vi "log analysis_gps.vi"() -> ()   [LabVIEW 2019] (continued)
0.0780,0.0969,0.1020,4.9076,0f000001,0*84139aa4\n\tsystem status\tnormal 2 27.900000 0 0\trobot status\t209.409703\t112.091356\t7.992300\t-0.536108\t-0.972920\t165.803914\t0.366000\t-0.087000\n\t\n15:41:04.9\tlog_raw\tgps_raw\t#INSPVAXA,USB3,0,46.5,FINESTEERING,2107,283282.900,02000000,471d,15824;INS_ALIGNMENT_COMPLETE,INS_RTKFIXED,37.37114058950,126.72319773387,7.9934,22.3000,0.0877,-0.2549,-0.0017,-0.494597000,-1.027505059,284.193699640,0.4479,0.2971,0.5695,0.1142,0.0928,0.0780,0.0969,0.1020,4.9076,0f000001,0*ecacd8f3\n\tsystem status\tnormal 2 27.900000 0 0\trobot status\t209.277787\t112.135444\t7.993400\t-0.494597\t-1.027505\t165.806300\t0.258000\t0.054000\n\t\n15:41:05.4\tlog_raw\tgps_raw\t\tsystem status\tnormal 2 27.900000 0 0\trobot status\t209.151815\t112.177150\t7.994600\t-0.569552\t-1.072991\t165.805716\t0.270000\t0.034000\n\t\n15:41:05.9\tlog_raw\tgps_raw\t\tsystem status\tnormal 2 27.900000 0 0\trobot status\t209.015709\t112.223223\t7.996800\t-0.645711\t-1.000745\t165.770418\t0.298000\t0.003000\n\t\n15:41:06.4\tlog_raw\tgps_raw\t#INSPVAXA,USB3,0,45.5,FINESTEERING,2107,283284.400,02000000,471d,15824;INS_ALIGNMENT_COMPLETE,INS_RTKFIXED,37.37114183564,126.72319312332,7.9966,22.3000,0.0813,-0.2603,0.0021,-0.541869353,-0.903555569,284.232610240,0.4477,0.2970,0.5694,0.1142,0.0928,0.0780,0.0969,0.1020,4.9102,0f000001,0*cca71bea\n\tsystem status\tnormal 2 27.900000 0 0\trobot status\t208.869392\t112.273757\t7.996600\t-0.541869\t-0.903556\t165.767390\t0.362000\t-0.089000\n\t\n15:41:06.9\tlog_raw\tgps_raw\t\tsystem status\tnormal 2 27.900000 0 0\trobot status\t208.748375\t112.316292\t7.995100\t-0.425843\t-0.804427\t165.786468\t0.277000\t0.029000\n\t\n15:41:07.4\tlog_raw\tgps_raw\t#INSPVAXA,USB3,0,48.5,FINESTEERING,2107,283285.400,02000000,471d,15824;INS_ALIGNMENT_COMPLETE,INS_RTKFIXED,37.37114271022,126.72319003823,7.9928,22.3000,0.0833,-0.2558,0.0046,-0.428723996,-1.048111002,284.209543070,0.4481,0.2971,0.5696,0.1142,0.0929,0.0780,0.0969,0.1020,4.9114,0f000001,0*c956834d\n\tsystem status\tnormal 2 27.900000 0 0\trobot status\t208.596120\t112.370829\t7.992800\t-0.428724\t-1.048111\t165.790457\t0.290000\t0.012000\n\t\n15:41:07.9\tlog_raw\tgps_raw\t\tsystem status\tnormal 2 27.900000 0 0\trobot status\t208.491998\t112.410695\t7.991800\t-0.503839\t-1.117557\t165.853585\t0.272000\t-0.014000\n\t\n15:41:08.4\tlog_raw\tgps_raw\t\tsystem status\tnormal 2 27.900000 0 0\trobot status\t208.354984\t112.461159\t7.990800\t-0.430331\t-1.222643\t165.896888\t0.242000\t0.064000\n\t\n15:41:08.9\tlog_raw\tgps_raw\t\tsystem status\tnormal 2 27.900000 0 0\trobot status\t208.213933\t112.512805\t7.989100\t-0.303789\t-1.363039\t165.889884\t0.281000\t0.011000\n\t\n15:41:09.4\tlog_raw\tgps_raw\t\tsystem status\tnormal 2 27.900000 0 0\trobot status\t208.079726\t112.560978\t7.988900\t-0.312448\t-1.099711\t166.040201\t0.268000\t0.063000\n\t\n15:41:09.9\tlog_raw\tgps_raw\t#INSPVAXA,USB3,0,48.5,FINESTEERING,2107,283287.900,02000000,471d,15824;INS_ALIGNMENT_COMPLETE,INS_RTKFIXED,37.37114488961,126.72318257858,7.9892,22.3000,0.0816,-0.2710,-0.0129,-0.307821910,-0.791572472,283.812578734,0.4475,0.2971,0.5695,0.1142,0.0928,0.0780,0.0969,0.1020,4.9139,0f000001,0*ad245747\n\tsystem status\tnormal 2 27.900000 0 0\trobot status\t207.935356\t112.612724\t7.989200\t-0.307822\t-0.791572\t166.187421\t0.253000\t0.089000\n\t\n15:41:10.4\tlog_raw\tgps_raw\t\tsystem status\tnormal 2 27.900000 0 0\trobot status\t207.818109\t112.654789\t7.987300\t-0.128529\t-0.454330\t166.386533\t0.238000\t0.094000\n\t\n15:41:10.9\tlog_raw\tgps_raw\t\tsystem status\tnormal 2 27.900000 0 0\trobot status\t207.682381\t112.702193\t7.985100\t0.008586\t-0.367132\t166.647704\t0.354000\t-0.072000\n\t\n15:41:11.4\tlog_raw\tgps_raw\t\tsystem status\tnormal 2 27.900000 0 0\trobot status\t207.545944\t112.748506\t7.983500\t-0.104519\t-0.407601\t166.876689\t0.236000\t0.094000\n\t\n15:41:11.9\tlog_raw\tgps_raw\t\tsystem status\tnormal 2 27.900000 0 0\trobot status\t207.410608\t112.793821\t7.982300\t-0.272687\t-0.577637\t167.093526\t0.359000\t-0.081000\n\t\n15:41:12.4\tlog_raw\tgps_raw\t#INSPVAXA,USB3,0,49.0,FINESTEERING,2107,283290.400,02000000,471d,15824;INS_ALIGNMENT_COMPLETE,INS_RTKFIXED,37.37114696201,126.72317494055,7.9797,22.3000,0.0686,-0.2611,-0.0031,-0.360570478,-0.610945799,282.620180984,0.4490,0.2972,0.5701,0.1142,0.0929,0.0781,0.0969,0.1020,4.9167,0f000001,0*1d53d3bd\n\tsystem status\tnormal 2 27.800000 0 0\trobot status\t207.258792\t112.842745\t7.979700\t-0.360570\t-0.610946\t167.379819\t0.257000\t0.055000\n\t\n15:41:12.9\tlog_raw\tgps_raw\t\tsystem status\tnormal 2 27.900000 0 0\trobot status\t207.133471\t112.884794\t7.976400\t-0.101922\t-0.587644\t167.621248\t0.377000\t-0.109000\n\t\n15:41:13.4\tlog_raw\tgps_raw\t#INSPVAXA,USB3,0,45.5,FINESTEERING,2107,283291.400,02000000,471d,15824;INS_ALIGNMENT_COMPLETE,INS_RTKFIXED,37.37114777556,126.72317182162,7.9735,22.3000,0.0763,-0.2712,-0.0094,-0.152974893,-0.616653887,282.239897550,0.4489,0.2971,0.5701,0.1142,0.0928,0.0781,0.0969,0.1020,4.9171,0f000001,0*c60dfbfa\n\tsystem status\tnormal 2 27.900000 0 0\trobot status\t206.982522\t112.933044\t7.973500\t-0.152975\t-0.616654\t167.760102\t0.226000\t0.111000\n\t\n15:41:13.9\tlog_raw\tgps_raw\t\tsystem status\tnormal 2 27.900000 0 0\trobot status\t206.858547\t112.972720\t7.970000\t-0.152145\t-0.757539\t167.961795\t0.320000\t-0.033000\n\t\n15:41:14.4\tlog_raw\tgps_raw\t\tsystem status\tnormal 2 27.900000 0 0\trobot status\t206.718471\t113.014805\t7.968100\t-0.313258\t-0.816536\t168.090661\t0.278000\t0.044000\n\t\n15:41:14.9\tlog_raw\tgps_raw\t#INSPVAXA,USB3,0,45.0,FINESTEERING,2107,283292.900,02008000,471d,15824;INS_ALIGNMENT_COMPLETE,INS_RTKFIXED,37.37114893041,126.72316711689,7.9673,22.3000,0.0793,-0.2669,-0.0229,-0.307538430,-0.866474135,281.723711903,0.4489,0.2972,0.5701,0.1141,0.0929,0.0781,0.0969,0.1020,4.9176,0f000001,0*1a68f6c8\n\tsystem status\tnormal 2 27.900000 0 0\trobot status\t206.565785\t113.061225\t7.967300\t-0.307538\t-0.866474\t168.276288\t0.236000\t0.105000\n\t\n15:41:15.4\tlog_raw\tgps_raw\t#INSPVAXA,USB3,0,46.5,FINESTEERING,2107,283293.400,02008000,471d,15824;INS_ALIGNMENT_COMPLETE,INS_RTKFIXED,37.37114931460,126.72316558102,7.9656,22.3000,0.0841,-0.2703,-0.0190,-0.304587768,-0.848212966,281.590040243,0.4485,0.2971,0.5701,0.1141,0.0929,0.0781,0.0969,0.1020,4.9184,0f000001,0*b7765035\n\tsystem status\tnormal 2 27.900000 0 0\trobot status\t206.429740\t113.103867\t7.965600\t-0.304588\t-0.848213\t168.409960\t0.206000\t0.139000\n\t\n15:41:15.9\tlog_raw\tgps_raw\t#INSPVAXA,USB3,0,46.5,FINESTEERING,2107,283293.900,02008000,471d,15824;INS_ALIGNMENT_COMPLETE,INS_RTKFIXED,37.37114971165,126.72316402474,7.9632,22.3000,0.0893,-0.2652,-0.0218,-0.263902472,-0.725819533,281.502254462,0.4485,0.2971,0.5701,0.1141,0.0929,0.0781,0.0969,0.1020,4.9184,0f000001,0*152a6832\n\tsystem status\tnormal 2 27.900000 0 0\trobot status\t206.291887\t113.147937\t7.963200\t-0.263902\t-0.725820\t168.497746\t0.243000\t0.082000\n\t\n15:41:16.4\tlog_raw\tgps_raw\t#DUALANTENNAHEADINGA,USB3,0,47.5,FINESTEERING,2107,283294.400,02008000,d426,15824;SOL_COMPUTED,L1_FLOAT,-1.000000000,239.844818115,64.606910706,0.0,166.616958618,114.780426025,\"631T\",14,7,7,7,04,00,20,23*19bdebe6\n\tsystem status\tnormal 2 27.900000 0 0\trobot status\t206.152884\t113.190709\t7.959900\t-0.163673\t-0.640565\t168.556497\t0.324000\t-0.032000\n\t\n15:41:16.9\tlog_raw\tgps_raw\t#INSPVAXA,USB3,0,47.5,FINESTEERING,2107,283294.900,02008000,471d,15824;INS_ALIGNMENT_COMPLETE,INS_RTKFIXED,37.37115047180,126.72316089302,7.9563,22.3000,0.0884,-0.2648,-0.0252,-0.144222363,-0.665231738,281.410020800,0.4483,0.2971,0.5702,0.1141,0.0929,0.0781,0.0969,0.1020,4.9194,0f000001,0*3b62bb88\n\tsystem status\tnormal 2 27.900000 0 0\trobot status\t206.014485\t113.232309\t7.956300\t-0.144222\t-0.665232\t168.589979\t0.247000\t0.081000\n\t\n15:41:17.4\tlog_raw\tgps_raw\t#INSPVAXA,USB3,0,50.0,FINESTEERING,2107,283295.400,02008000,471d,15824;INS_ALIGNMENT_COMPLETE,INS_RTKFIXED,37.37115084282,126.72315933978,7.9528,22.3000,0.0924,-0.2759,-0.0196,-0.193072423,-0.599159987,281.404191398,0.4483,0.2972,0.5704,0.1141,0.0929,0.0781,0.0969,0.1020,4.9206,0f000001,0*10d0b358\n\tsystem status\tnormal 2 27.900000 0 0\trobot status\t205.876901\t113.273490\t7.952800\t-0.193072\t-0.599160\t168.595809\t0.232000\t0.099000\n\t\n15:41:17.9\tlog_raw\tgps_raw\t#DUALANTENNAHEADINGA,USB3,0,50.0,FINESTEERING,2107,283295.900,02008000,d426,15824;SOL_COMPUTED,L1_FLOAT,-1.000000000,237.505355835,63.904857635,0.0,132.502212524,100.132637024,\"631T\",18,7,7,7,04,00,20,23*65892cbe\n\tsystem status\tnormal 2 27.900000 0 0\trobot status\t205.736785\t113.315150\t7.949200\t-0.260802\t-0.582967\t168.632293\t0.363000\t-0.102000\n\t\n15:41:18.4\tlog_raw\tgps_raw\t#INSPVAXA,USB3,0,48.0,FINESTEERING,2107,283296.400,02000000,471d,15824;INS_ALIGNMENT_COMPLETE,INS_RTKFIXED,37.37115159718,126.72315615738,7.9465,22.3000,0.0791,-0.2694,-0.0207,-0.243399064,-0.670303130,281.350381615,0.4482,0.2972,0.5704,0.1141,0.0929,0.0781,0.0969,0.1020,4.9219,0f000001,0*42d4064f\n\tsystem status\tnormal 2 27.900000 0 0\trobot status\t205.595010\t113.357219\t7.946500\t-0.243399\t-0.670303\t168.649618\t0.251000\t0.069000\n\t\n15:41:18.9\tlog_raw\tgps_raw\t#DUALANTENNAHEADINGA,USB3,0,48.0,FINESTEERING,2107,283296.900,02000000,d426,15824;SOL_COMPUTED,L1_FLOAT,-1.000000000,239.343627930,64.402900696,0.0,148.477706909,103.162033081,\"631T\",15,7,7,7,04,00,20,23*e8ad3b91\n\tsystem status\tnormal 2 27.900000 0 0\trobot status\t205.455731\t113.398696\t7.943200\t-0.247026\t-0.834415\t168.640311\t0.263000\t0.052000\n\t\n15:41:19.4\tlog_raw\tgps_raw\t#INSPVAXA,USB3,0,48.5,FINESTEERING,2107,283297.400,02000000,471d,15824;INS_ALIGNMENT_COMPLETE,INS_RTKFIXED,37.37115233691,126.72315301561,7.9394,22.3000,0.0884,-0.2678,-0.0159,-0.231727201,-0.925475232,281.406187486,0.4479,0.2972,0.5705,0.1141,0.0929,0.0781,0.0969,0.1020,4.9234,0f000001,0*12bb3ab8\n\tsystem status\tnormal 2 27.900000 0 0\trobot status\t205.316717\t113.439324\t7.939400\t-0.231727\t-0.925475\t168.593813\t0.254000\t0.056000\n\t\n15:41:19.9\tlog_raw\tgps_raw\t#INSPVAXA,USB3,0,48.5,FINESTEERING,2107,283297.900,02000000,471d,15824;INS_ALIGNMENT_COMPLETE,INS_RTKFIXED,37.37115269099,126.72315144073,7.9365,22.3000,0.0910,-0.2656,-0.0151,-0.313313206,-1.052318867,281.426390145,0.4479,0.2972,0.5705,0.1141,0.0929,0.0781,0.0969,0.1020,4.9234,0f000001,0*736ed8bf\n\tsystem status\tnormal 2 27.900000 0 0\trobot status\t205.177217\t113.478625\t7.936500\t-0.313313\t-1.052319\t168.573610\t0.338000\t-0.064000\n\t\n15:41:20.4\tlog_raw\tgps_raw\t#INSPVAXA,USB3,0,51.0,FINESTEERING,2107,283298.400,02008000,471d,15824;INS_ALIGNMENT_COMPLETE,INS_RTKFIXED,37.37115305235,126.72314988342,7.9353,22.3000,0.0916,-0.2769,-0.0209,-0.334551062,-1.062649728,281.510450762,0.4462,0.2970,0.5704,0.1139,0.0928,0.0781,0.0969,0.1019,4.9249,0f000001,0*7ea0d7b1\n\tsystem status\tnormal 2 27.900000 0 0\trobot status\t205.039273\t113.518734\t7.935300\t-0.334551\t-1.062650\t168.489549\t0.305000\t-0.007000\n\t\n15:41:20.9\tlog_raw\tgps_raw\t#INSPVAXA,USB3,0,51.0,FINESTEERING,2107,283298.900,02008000,471d,15824;INS_ALIGNMENT_COMPLETE,INS_RTKFIXED,37.37115341393,126.72314832428,7.9330,22.3000,0.0837,-0.2625,-0.0169,-0.397478234,-1.037439092,281.585618235,0.4462,0.2970,0.5704,0.1139,0.0928,0.0781,0.0969,0.1019,4.9249,0f000001,0*addaa3c1\n\tsystem status\tnormal 2 27.900000 0 0\trobot status\t204.901166\t113.558867\t7.933000\t-0.397478\t-1.037439\t168.414382\t0.285000\t0.002000\n\t\n15:41:21.4\tlog_raw\tgps_raw\t#INSPVAXA,USB3,0,45.0,FINESTEERING,2107,283299.400,02008000,471d,15824;INS_ALIGNMENT_COMPLETE,INS_RTKFIXED,37.37115377370,126.72314676184,7.9298,22.3000,0.0909,-0.2631,-0.0145,-0.362966216,-0.969827593,281.677827339,0.4450,0.2970,0.5703,0.1138,0.0928,0.0781,0.0969,0.1019,4.9264,0f000001,0*1c473296\n\tsystem status\tnormal 2 27.900000 0 0\trobot status\t204.762768\t113.598800\t7.929800\t-0.362966\t-0.969828\t168.322173\t0.292000\t-0.002000\n\t\n15:41:21.9\tlog_raw\tgps_raw\t#INSPVAXA,USB3,0,45.0,FINESTEERING,2107,283299.900,02008000,471d,15824;INS_ALIGNMENT_COMPLETE,INS_RTKFIXED,37.37115412853,126.72314521703,7.9265,22.3000,0.0831,-0.2721,-0.0168,-0.334055092,-0.857613920,281.755753897,0.4450,0.2970,0.5703,0.1138,0.0928,0.0781,0.0969,0.1019,4.9264,0f000001,0*4d7a0a60\n\tsystem status\tnormal 2 27.900000 0 0\trobot status\t204.625931\t113.638184\t7.926500\t-0.334055\t-0.857614\t168.244246\t0.298000\t-0.006000\n\t\n15:41:22.4\tlog_raw\tgps_raw\t#DUALANTENNAHEADINGA,USB3,0,40.5,FINESTEERING,2107,283300.400,02008000,d426,15824;SOL_COMPUTED,L1_FLOAT,-1.000000000,232.358734131,64.946899414,0.0,184.697021484,151.855468750,\"631T\",13,5,5,5,04,00,20,03*f60c6ef8\n\tsystem status\tnormal 2 27.900000 0 0\trobot status\t204.490325\t113.677128\t7.923100\t-0.506518\t-0.923731\t168.214160\t0.298000\t-0.006000\n\t\n15:41:22.9\tlog_raw\tgps_raw\t#INSPVAXA,USB3,0,40.5,FINESTEERING,2107,283300.900,02008000,471d,15824;INS_ALIGNMENT_COMPLETE,INS_RTKFIXED,37.37115484988,126.72314211300,7.9189,22.3000,0.0947,-0.2610,-0.0185,-0.569818245,-0.847887628,281.897603844,0.4441,0.2969,0.5702,0.1137,0.0928,0.0781,0.0969,0.1019,4.9278,0f000001,0*956f8967\n\tsystem status\tnormal 2 27.900000 0 0\trobot status\t204.350981\t113.718249\t7.918900\t-0.569818\t-0.847888\t168.102396\t0.293000\t0.000000\n\t\n15:41:23.4\tlog_raw\tgps_raw\t#DUALANTENNAHEADINGA,USB3,0,48.5,FINESTEERING,2107,283301.400,02008000,d426,15824;SOL_COMPUTED,L1_FLOAT,-1.000000000,241.477539063,62.723838806,0.0,360.000000000,180.000000000,\"631T\",17,6,6,5,04,00,20,03*c892e55f\n\tsystem status\tnormal 2 28.000000 0 0\trobot status\t204.213454\t113.758293\t7.915500\t-0.559323\t-0.799162\t167.987506\t0.300000\t-0.003000\n\t\n15:41:23.9\tlog_raw\tgps_raw\t#INSPVAXA,USB3,0,48.5,FINESTEERING,2107,283301.900,02008000,471d,15824;INS_ALIGNMENT_COMPLETE,INS_RTKFIXED,37.37115557070,126.72313902980,7.9130,22.3000,0.0918,-0.2789,-0.0166,-0.521820330,-0.769982441,282.107376455,0.4435,0.2967,0.5700,0.1137,0.0928,0.0780,0.0969,0.1019,4.9292,0f000001,0*6ce7102f\n\tsystem status\tnormal 2 27.900000 0 0\trobot status\t204.077877\t113.798256\t7.913000\t-0.521820\t-0.769982\t167.892624\t0.298000\t-0.006000\n\t\n15:41:24.4\tlog_raw\tgps_raw\t#DUALANTENNAHEADINGA,USB3,0,45.0,FINESTEERING,2107,283302.400,02000000,d426,15824;SOL_COMPUTED,NARROW_FLOAT,-1.000000000,244.334762573,52.398559570,0.0,117.969345093,144.888336182,\"631T\",16,7,7,5,04,00,20,03*fc904e6e\n\tsystem status\tnormal 2 27.900000 0 0\trobot status\t203.939790\t113.838541\t7.911100\t-0.641899\t-0.763292\t167.767932\t0.296000\t-0.008000\n\t\n15:41:24.9\tlog_raw\tgps_raw\t#INSPVAXA,USB3,0,45.0,FINESTEERING,2107,283302.900,02000000,471d,15824;INS_ALIGNMENT_COMPLETE,INS_RTKFIXED,37.37115630629,126.72313591072,7.9093,22.3000,0.0953,-0.2572,-0.0206,-0.734868451,-0.639941335,282.297303712,0.4435,0.2967,0.5699,0.1137,0.0928,0.0780,0.0969,0.1019,4.9307,0f000001,0*e76bd6df\n\tsystem status\tnormal 2 27.900000 0 0\trobot status\t203.801594\t113.879902\t7.909300\t-0.734868\t-0.639941\t167.702696\t0.294000\t-0.003000\n\t\n15:41:25.4\tlog_raw\tgps_raw\t#DUALANTENNAHEADINGA,USB3,0,47.0,FINESTEERING,2107,283303.400,02000000,d426,15824;SOL_COMPUTED,NARROW_FLOAT,-1.000000000,231.882415771,63.058189392,0.0,139.197525024,151.772613525,\"631T\",16,5,5,5,04,00,20,03*97a548ee\n\tsystem status\tnormal 2 27.900000 0 0\trobot status\t203.663374\t113.921399\t7.906600\t-0.772718\t-0.613063\t167.570919\t0.302000\t-0.004000\n\t\n15:41:25.9\tlog_raw\tgps_raw\t#DUALANTENNAHEADINGA,USB3,0,47.0,FINESTEERING,2107,283303.900,02000000,d426,15824;SOL_COMPUTED,NARROW_FLOAT,-1.000000000,232.017898560,63.345188141,0.0,143.997665405,156.088058472,\"631T\",16,5,5,5,04,00,20,03*4eb7c41d\n\tsystem status\tnormal 2 27.900000 0 0\trobot status\t203.531143\t113.962488\t7.903700\t-0.724838\t-0.600156\t167.494385\t0.294000\t-0.010000\n\t\n15:41:26.4\tlog_raw\tgps_raw\t#DUALANTENNAHEADINGA,USB3,0,48.5,FINESTEERING,2107,283304.400,02000000,d426,15824;SOL_COMPUTED,NARROW_FLOAT,-1.000000000,234.068984985,56.849258423,0.0,140.735427856,121.552192688,\"631T\",17,5,5,5,04,00,20,03*01bf1f6c\n\tsystem status\tnormal 2 28.000000 0 0\trobot status\t203.391424\t114.004312\t7.901000\t-0.774710\t-0.760867\t167.345105\t0.295000\t0.000000\n\t\n15:41:26.9\tlog_raw\tgps_raw\t#DUALANTENNAHEADINGA,USB3,0,48.5,FINESTEERING,2107,283304.900,02000000,d426,15824;SOL_COMPUTED,NARROW_FLOAT,-1.000000000,233.255889893,60.512351990,0.0,144.115737915,132.290557861,\"631T\",16,5,5,5,04,00,20,03*f75e5353\n\tsystem status\tnormal 2 28.000000 0 0\trobot status\t203.253011\t114.046330\t7.898300\t-0.773429\t-0.872963\t167.221831\t0.303000\t0.000000\n\t\n15:41:27.4\tlog_raw\tgps_raw\t#DUALANTENNAHEADINGA,USB3,0,44.5,FINESTEERING,2107,283305.400,02000000,d426,15824;SOL_COMPUTED,L1_FLOAT,-1.000000000,233.577301025,62.029331207,0.0,96.220359802,93.397712708,\"631T\",16,7,7,7,04,00,20,23*c706f208\n\tsystem status\tnormal 2 27.900000 0 0\trobot status\t203.115679\t114.089504\t7.895500\t-0.788524\t-0.978908\t167.126035\t0.304000\t-0.003000\n\t\n15:41:27.9\tlog_raw\tgps_raw\t#INSPVAXA,USB3,0,44.5,FINESTEERING,2107,283305.900,02000000,471d,15824;INS_ALIGNMENT_COMPLETE,INS_RTKFIXED,37.37115859876,126.72312661710,7.8931,22.3000,0.1099,-0.2740,-0.0203,-0.656948256,-1.026367875,282.954540739,0.4425,0.2966,0.5699,0.1135,0.0928,0.0781,0.0969,0.1019,4.9352,0f000001,0*1036819f\n\tsystem status\tnormal 2 27.900000 0 0\trobot status\t202.978380\t114.134351\t7.893100\t-0.656948\t-1.026368\t167.045459\t0.302000\t-0.002000\n\t\n15:41:28.4\tlog_raw\tgps_raw\t#INSPVAXA,USB3,0,46.0,FINESTEERING,2107,283306.400,02000000,471d,15824;INS_ALIGNMENT_COMPLETE,INS_RTKFIXED,37.37115900607,126.72312505339,7.8906,22.3000,0.1023,-0.2590,-0.0088,-0.729755856,-0.991327680,283.031299581,0.4419,0.2965,0.5696,0.1135,0.0928,0.0780,0.0969,0.1019,4.9367,0f000001,0*5e887597\n\tsystem status\tnormal 2 27.900000 0 0\trobot status\t202.839869\t114.179559\t7.890600\t-0.729756\t-0.991328\t166.968700\t0.296000\t-0.004000\n\t\n15:41:28.9\tlog_raw\tgps_raw\t#DUALANTENNAHEADINGA,USB3,0,46.0,FINESTEERING,2107,283306.900,02000000,d426,15824;SOL_COMPUTED,L1_FLOAT,-1.000000000,239.290145874,67.008094788,0.0,195.596420288,134.664169312,\"631T\",14,5,5,5,04,00,20,03*267cdbf0\n\tsystem status\tnormal 2 27.900000 0 0\trobot status\t202.702346\t114.224740\t7.887600\t-0.783555\t-0.902622\t166.912380\t0.303000\t-0.003000\n\t\n15:41:29.4\tlog_raw\tgps_raw\t#DUALANTENNAHEADINGA,USB3,0,49.5,FINESTEERING,2107,283307.400,02000000,d426,15824;SOL_COMPUTED,L1_FLOAT,-1.000000000,232.261947632,66.446723938,0.0,159.915008545,144.811691284,\"631T\",14,5,5,5,04,00,20,03*cd69fe68\n\tsystem status\tnormal 2 27.900000 0 0\trobot status\t202.568399\t114.268173\t7.884600\t-0.734963\t-0.759541\t166.891334\t0.256000\t0.056000\n\t\n15:41:29.9\tlog_raw\tgps_raw\t#DUALANTENNAHEADINGA,USB3,0,49.5,FINESTEERING,2107,283307.900,02000000,d426,15824;SOL_COMPUTED,L1_FLOAT,-1.000000000,232.562942505,64.960189819,0.0,154.937866211,134.466018677,\"631T\",15,5,5,5,04,00,20,03*e7f8f672\n\tsystem status\tnormal 2 27.900000 0 0\trobot status\t202.433799\t114.310718\t7.881800\t-0.734495\t-0.652410\t166.951453\t0.361000\t-0.092000\n\t\n15:41:30.4\tlog_raw\tgps_raw\t#DUALANTENNAHEADINGA,USB3,0,51.0,FINESTEERING,2107,283308.400,02000000,d426,15824;SOL_COMPUTED,L1_FLOAT,-1.000000000,235.060028076,63.952377319,0.0,259.231262207,169.746810913,\"631T\",15,5,5,5,04,00,20,03*f7293e70\n\tsystem status\tnormal 2 27.900000 0 0\trobot status\t202.297404\t114.353381\t7.879900\t-0.750628\t-0.536234\t166.976163\t0.281000\t0.025000\n\t\n15:41:30.9\tlog_raw\tgps_raw\t#INSPVAXA,USB3,0,51.0,FINESTEERING,2107,283308.900,02000000,471d,15824;INS_ALIGNMENT_COMPLETE,INS_RTKFIXED,37.37116096041,126.72311737455,7.8778,22.3000,0.0846,-0.2672,-0.0151,-0.781249790,-0.507158310,282.995006932,0.4410,0.2964,0.5694,0.1133,0.0927,0.0780,0.0968,0.1018,4.9395,0f000001,0*4118e416\n\tsystem status\tnormal 2 27.900000 0 0\trobot status\t202.159690\t114.396477\t7.877800\t-0.781250\t-0.507158\t167.004993\t0.286000\t0.019000\n\t\n15:41:31.4\tlog_raw\tgps_raw\t#INSPVAXA,USB3,0,47.5,FINESTEERING,2107,283309.400,02000000,471d,15824;INS_ALIGNMENT_COMPLETE,INS_RTKFIXED,37.37116135505,126.72311582888,7.8756,22.3000,0.0948,-0.2836,-0.0131,-0.715867261,-0.524623551,282.915298910,0.4409,0.2962,0.5692,0.1133,0.0927,0.0780,0.0968,0.1018,4.9410,0f000001,0*81cbe5cb\n\tsystem status\tnormal 2 27.900000 0 0\trobot status\t202.022777\t114.440279\t7.875600\t-0.715867\t-0.524624\t167.084701\t0.380000\t-0.117000\n\t\n15:41:31.9\tlog_raw\tgps_raw\t#INSPVAXA,USB3,0,47.5,FINESTEERING,2107,283309.900,02000000,471d,15824;INS_ALIGNMENT_COMPLETE,INS_RTKFIXED,37.37116173975,126.72311427706,7.8728,22.3000,0.0962,-0.2788,-0.0165,-0.819724442,-0.652921379,282.793511775,0.4409,0.2962,0.5692,0.1133,0.0927,0.0780,0.0968,0.1018,4.9410,0f000001,0*d0f32b82\n\tsystem status\tnormal 2 27.900000 0 0\trobot status\t201.885319\t114.482979\t7.872800\t-0.819724\t-0.652921\t167.206488\t0.287000\t0.021000\n\t\n15:41:32.4\tlog_raw\tgps_raw\t#DUALANTENNAHEADINGA,USB3,0,49.5,FINESTEERING,2107,283310.400,02000000,d426,15824;SOL_COMPUTED,NARROW_FLOAT,-1.000000000,251.362304688,59.888744354,0.0,206.856552124,155.140167236,\"631T\",17,7,7,5,04,00,20,03*1094d047\n\tsystem status\tnormal 2 27.900000 0 0\trobot status\t201.748050\t114.524563\t7.870500\t-0.938813\t-0.746948\t167.374940\t0.246000\t0.082000\n\t\n15:41:32.9\tlog_raw\tgps_raw\t#DUALANTENNAHEADINGA,USB3,0,49.5,FINESTEERING,2107,283310.900,02000000,d426,15824;SOL_COMPUTED,NARROW_FLOAT,-1.000000000,251.351150513,59.773147583,0.0,206.432357788,155.578613281,\"631T\",16,7,7,5,04,00,20,03*7af03570\n\tsystem status\tnormal 2 27.900000 0 0\trobot status\t201.610292\t114.567045\t7.868700\t-0.871424\t-0.892330\t167.536678\t0.323000\t-0.031000\n\t\n15:41:33.4\tlog_raw\tgps_raw\t#INSPVAXA,USB3,0,48.0,FINESTEERING,2107,283311.400,02000000,471d,15824;INS_ALIGNMENT_COMPLETE,INS_RTKFIXED,37.37116288417,126.72310962036,7.8652,22.3000,0.0869,-0.2743,-0.0174,-0.761855040,-0.888417271,282.272425942,0.4407,0.2962,0.5691,0.1131,0.0927,0.0780,0.0968,0.1018,4.9438,0f000001,0*0cfd0bf9\n\tsystem status\tnormal 2 27.900000 0 0\trobot status\t201.472837\t114.610001\t7.865200\t-0.761855\t-0.888417\t167.727574\t0.245000\t0.089000\n\t\n15:41:33.9\tlog_raw\tgps_raw\t#DUALANTENNAHEADINGA,USB3,0,48.0,FINESTEERING,2107,283311.900,02000000,d426,15824;SOL_COMPUTED,NARROW_FLOAT,-1.000000000,256.476898193,63.091281891,0.0,360.000000000,180.000000000,\"631T\",16,6,6,5,04,00,20,03*76034569\n\tsystem status\tnormal 2 27.900000 0 0\trobot status\t201.335540\t114.653174\t7.860100\t-0.684071\t-1.038231\t167.853976\t0.342000\t-0.072000\n\t\n15:41:34.4\tlog_raw\tgps_raw\t#DUALANTENNAHEADINGA,USB3,0,47.0,FINESTEERING,2107,283312.400,02000000,d426,15824;SOL_COMPUTED,L1_FLOAT,-1.000000000,236.672042847,63.326492310,0.0,146.049911499,114.689262390,\"631T\",17,5,5,5,04,00,20,03*2d6dda53\n\tsystem status\tnormal 2 27.900000 0 0\trobot status\t201.199331\t114.694596\t7.855800\t-0.737324\t-1.007911\t167.998905\t0.207000\t0.142000\n\t\n15:41:34.9\tlog_raw\tgps_raw\t#DUALANTENNAHEADINGA,USB3,0,47.0,FINESTEERING,2107,283312.900,02000000,d426,15824;SOL_COMPUTED,L1_FLOAT,-1.000000000,236.406433105,63.618362427,0.0,144.065521240,114.259201050,\"631T\",19,5,5,5,04,00,20,03*a0545f5a\n\tsystem status\tnormal 2 27.900000 0 0\trobot status\t201.061886\t114.736958\t7.852100\t-0.673596\t-0.901081\t168.144481\t0.395000\t-0.123000\n\t\n15:41:35.4\tlog_raw\tgps_raw\t#DUALANTENNAHEADINGA,USB3,0,48.0,FINESTEERING,2107,283313.400,02000000,d426,15824;SOL_COMPUTED,NARROW_FLOAT,-1.000000000,249.966949463,62.680927277,0.0,300.232086182,155.331420898,\"631T\",19,8,8,6,04,00,20,23*b56427c2\n\tsystem status\tnormal 2 27.900000 0 0\trobot status\t200.925110\t114.778837\t7.848800\t-0.630597\t-0.967997\t168.265961\t0.270000\t0.054000\n\t\n15:41:35.9\tlog_raw\tgps_raw\t#DUALANTENNAHEADINGA,USB3,0,48.0,FINESTEERING,2107,283313.900,02000000,d426,15824;SOL_COMPUTED,NARROW_FLOAT,-1.000000000,249.735733032,62.666515350,0.0,296.963775635,155.122772217,\"631T\",17,8,8,7,04,00,20,23*38c36f09\n\tsystem status\tnormal 2 27.900000 0 0\trobot status\t200.813052\t114.814862\t7.843800\t-0.601513\t-0.911436\t168.475071\t0.337000\t-0.013000\n\t\n15:41:36.4\tlog_raw\tgps_raw\t#DUALANTENNAHEADINGA,USB3,0,48.0,FINESTEERING,2107,283314.400,02000000,d426,15824;SOL_COMPUTED,L1_FLOAT,-1.000000000,262.029388428,61.695976257,0.0,360.000000000,162.501907349,\"631T\",16,8,8,7,04,00,20,23*1cdc20bd\n\tsystem status\tnormal 2 27.900000 0 0\trobot status\t200.674190\t114.856511\t7.838600\t-0.527796\t-0.888572\t168.515964\t0.278000\t0.017000\n\t\n15:41:36.9\tlog_raw\tgps_raw\t#DUALANTENNAHEADINGA,USB3,0,48.0,FINESTEERING,2107,283314.900,02000000,d426,15824;SOL_COMPUTED,L1_FLOAT,-1.000000000,261.856536865,61.556816101,0.0,360.000000000,163.368423462,\"631T\",15,8,8,7,04,00,20,23*198a35c5\n\tsystem status\tnormal 2 27.900000 0 0\trobot status\t200.535349\t114.897383\t7.834300\t-0.483100\t-0.849642\t168.578759\t0.284000\t0.007000\n\t\n15:41:37.4\tlog_raw\tgps_raw\t#DUALANTENNAHEADINGA,USB3,0,49.0,FINESTEERING,2107,283315.400,02000000,d426,15824;SOL_COMPUTED,L1_FLOAT,-1.000000000,241.071945190,70.013267517,0.0,216.117965698,130.788757324,\"631T\",14,7,7,7,04,00,20,23*ac92fc81\n\tsystem status\tnormal 2 27.900000 0 0\trobot status\t200.396113\t114.939229\t7.831400\t-0.323383\t-0.807085\t168.587932\t0.292000\t0.003000\n\t\n15:41:37.9\tlog_raw\tgps_raw\t#DUALANTENNAHEADINGA,USB3,0,49.0,FINESTEERING,2107,283315.900,02000000,d426,15824;SOL_COMPUTED,L1_FLOAT,-1.000000000,240.838073730,70.253372192,0.0,215.071411133,130.065658569,\"631T\",14,7,7,7,04,00,20,23*360ed7d2\n\tsystem status\tnormal 2 27.900000 0 0\trobot status\t200.260871\t114.980760\t7.828400\t-0.157937\t-0.664685\t168.654276\t0.256000\t0.067000\n\t\n15:41:38.4\tlog_raw\tgps_raw\t#DUALANTENNAHEADINGA,USB3,0,50.0,FINESTEERING,2107,283316.400,02000000,d426,15824;SOL_COMPUTED,L1_FLOAT,-1.000000000,243.607940674,69.715850830,0.0,272.601806641,140.221450806,\"631T\",14,7,7,7,04,00,20,23*51c69ef2\n\tsystem status\tnormal 2 27.900000 0 0\trobot status\t200.124189\t115.021827\t7.824500\t-0.144451\t-0.563579\t168.722514\t0.265000\t0.064000\n\t\n15:41:38.9\tlog_raw\tgps_raw\t#DUALANTENNAHEADINGA,USB3,0,50.0,FINESTEERING,2107,283316.900,02000000,d426,15824;SOL_COMPUTED,L1_FLOAT,-1.000000000,245.043029785,68.131629944,0.0,281.695404053,144.677200317,\"631T\",15,7,7,7,04,00,20,23*f1a17a24\n\tsystem status\tnormal 2 27.900000 0 0\trobot status\t199.986933\t115.062817\t7.821200\t-0.245938\t-0.522562\t168.786697\t0.289000\t0.018000\n\t\n15:41:39.4\tlog_raw\tgps_raw\t#DUALANTENNAHEADINGA,USB3,0,50.0,FINESTEERING,2107,283317.400,02000000,d426,15824;SOL_COMPUTED,L1_FLOAT,-1.000000000,270.938415527,64.219497681,0.0,360.000000000,166.916473389,\"631T\",15,8,8,7,04,00,20,23*09ee87ba\n\tsystem status\tnormal 2 27.900000 0 0\trobot status\t199.848763\t115.104066\t7.818400\t-0.204742\t-0.525836\t168.810423\t0.287000\t0.014000\n\t\n15:41:39.9\tlog_raw\tgps_raw\t#DUALANTENNAHEADINGA,USB3,0,50.0,FINESTEERING,2107,283317.900,02000000,d426,15824;SOL_COMPUTED,L1_FLOAT,-1.000000000,270.609985352,63.750827789,0.0,360.000000000,169.041946411,\"631T\",17,8,8,7,04,00,20,23*f5bf3eac\n\tsystem status\tnormal 2 27.900000 0 0\trobot status\t199.711437\t115.145257\t7.816200\t-0.090343\t-0.545239\t168.866636\t0.296000\t0.012000\n\t\n15:41:40.4\tlog_raw\tgps_raw\t#DUALANTENNAHEADINGA,USB3,0,47.5,FINESTEERING,2107,283318.400,02000000,d426,15824;SOL_COMPUTED,NARROW_FLOAT,-1.000000000,281.381378174,66.745414734,0.0,360.000000000,168.558471680,\"631T\",17,8,8,7,04,00,20,23*c33407f9\n\tsystem status\tnormal 2 27.900000 0 0\trobot status\t199.574384\t115.185773\t7.815400\t-0.137298\t-0.530182\t168.895194\t0.372000\t-0.108000\n\t\n15:41:40.9\tlog_raw\tgps_raw\t#DUALANTENNAHEADINGA,USB3,0,47.5,FINESTEERING,2107,283318.900,02000000,d426,15824;SOL_COMPUTED,NARROW_FLOAT,-1.000000000,279.926574707,66.934852600,0.0,360.000000000,167.527023315,\"631T\",17,8,8,7,04,00,20,23*f3d388f9\n\tsystem status\tnormal 2 27.900000 0 0\trobot status\t199.437201\t115.227141\t7.814900\t-0.190947\t-0.484012\t168.896184\t0.281000\t0.022000\n\t\n15:41:41.4\tlog_raw\tgps_raw\t#DUALANTENNAHEADINGA,USB3,0,45.0,FINESTEERING,2107,283319.400,02000000,d426,15824;SOL_COMPUTED,L1_FLOAT,-1.000000000,249.257110596,70.348373413,0.0,326.773925781,134.559478760,\"631T\",16,7,7,7,04,00,20,23*e6bdd1ed\n\tsystem status\tnormal 2 27.900000 0 0\trobot status\t199.297850\t115.268857\t7.814900\t-0.138877\t-0.515163\t168.909065\t0.268000\t0.032000\n\t\n15:41:41.9\tlog_raw\tgps_raw\t#DUALANTENNAHEADINGA,USB3,0,45.0,FINESTEERING,2107,283319.900,02000000,d426,15824;SOL_COMPUTED,L1_FLOAT,-1.000000000,248.767288208,70.954589844,0.0,326.445281982,135.310943604,\"631T\",14,5,5,5,04,00,20,03*3a82e8e8\n\tsystem status\tnormal 2 27.900000 0 0\trobot status\t199.156447\t115.310701\t7.815400\t-0.158989\t-0.594408\t168.944358\t0.297000\t0.013000\n\t\n15:41:42.4\tlog_raw\tgps_raw\t#DUALANTENNAHEADINGA,USB3,0,46.5,FINESTEERING,2107,283320.400,02000000,d426,15824;SOL_COMPUTED,L1_FLOAT,-1.000000000,258.042144775,75.598983765,0.0,360.000000000,180.000000000,\"631T\",15,5,5,5,04,00,20,03*b6617cb0\n\tsystem status\tnormal 2 27.900000 0 0\trobot status\t199.016475\t115.351763\t7.814800\t-0.357583\t-0.675596\t168.972205\t0.251000\t0.076000\n\t\n15:41:42.9\tlog_raw\tgps_raw\t#DUALANTENNAHEADINGA,USB3,0,46.5,FINESTEERING,2107,283320.900,02000000,d426,15824;SOL_COMPUTED,L1_FLOAT,-1.000000000,253.391662598,75.137130737,0.0,360.000000000,180.000000000,\"631T\",14,5,5,5,04,00,20,03*50d197fe\n\tsystem status\tnormal 2 27.900000 0 0\trobot status\t198.877003\t115.393675\t7.813600\t-0.439418\t-0.704299\t168.953352\t0.349000\t-0.082000\n\t\n15:41:43.4\tlog_raw\tgps_raw\t#DUALANTENNAHEADINGA,USB3,0,46.5,FINESTEERING,2107,283321.400,02000000,d426,15824;SOL_COMPUTED,L1_FLOAT,-1.000000000,312.583312988,56.468681335,0.0,360.000000000,180.000000000,\"631T\",14,6,6,5,04,00,20,03*0f80647d\n\tsystem status\tnormal 2 27.900000 0 0\trobot status\t198.736520\t115.435996\t7.812200\t-0.475385\t-0.762357\t168.980810\t0.355000\t-0.086000\n\t\n15:41:43.9\tlog_raw\tgps_raw\t#DUALANTENNAHEADINGA,USB3,0,46.5,FINESTEERING,2107,283321.900,02000000,d426,15824;SOL_COMPUTED,L1_FLOAT,-1.000000000,310.554901123,55.892704010,0.0,360.000000000,180.000000000,\"631T\",16,6,6,5,04,00,20,03*74537864\n\tsystem status\tnormal 2 27.900000 0 0\trobot status\t198.596710\t115.478140\t7.811100\t-0.557068\t-0.791255\t168.983949\t0.262000\t0.047000\n\t\n15:41:44.4\tlog_raw\tgps_raw\t#DUALANTENNAHEADINGA,USB3,0,41.0,FINESTEERING,2107,283322.400,02008000,d426,15824;SOL_COMPUTED,L1_FLOAT,-1.000000000,241.266906738,69.189468384,0.0,360.000000000,180.000000000,\"631T\",17,5,5,5,04,00,20,03*c679f6f8\n\tsystem status\tnormal 2 27.900000 0 0\trobot status\t198.456995\t115.521016\t7.808800\t-0.575238\t-0.758835\t168.989288\t0.328000\t-0.051000\n\t\n15:41:44.9\tlog_raw\tgps_raw\t#DUALANTENNAHEADINGA,USB3,0,41.0,FINESTEERING,2107,283322.900,02008000,d426,15824;SOL_COMPUTED,L1_FLOAT,-1.000000000,239.202957153,73.481590271,0.0,360.000000000,180.000000000,\"631T\",16,5,5,5,04,00,20,03*1cc6a146\n\tsystem status\tnormal 2 27.900000 0 0\trobot status\t198.315403\t115.564555\t7.806200\t-0.625577\t-0.773974\t168.969066\t0.282000\t0.024000\n\t\n15:41:45.4\tlog_raw\tgps_raw\t#DUALANTENNAHEADINGA,USB3,0,47.5,FINESTEERING,2107,283323.400,02008000,d426,15824;SOL_COMPUTED,L1_FLOAT,-1.000000000,238.744445801,53.518810272,0.0,151.505752563,125.381988525,\"631T\",19,6,6,5,04,00,20,03*673b97e4\n\tsystem status\tnormal 2 27.900000 0 0\trobot status\t198.173933\t115.605465\t7.804400\t-0.715732\t-0.866994\t168.992005\t0.365000\t-0.095000\n\t\n15:41:45.9\tlog_raw\tgps_raw\t#DUALANTENNAHEADINGA,USB3,0,47.5,FINESTEERING,2107,283323.900,02008000,d426,15824;SOL_COMPUTED,L1_FLOAT,-1.000000000,240.007232666,54.498615265,0.0,179.365921021,137.099334717,\"631T\",17,6,6,5,04,00,20,03*8af523f5\n\tsystem status\tnormal 2 27.900000 0 0\trobot status\t198.031198\t115.646553\t7.802300\t-0.784626\t-0.855165\t169.011485\t0.286000\t0.025000\n\t\n15:41:46.4\tlog_raw\tgps_raw\t#DUALANTENNAHEADINGA,USB3,0,45.5,FINESTEERING,2107,283324.400,02008000,d426,15824;SOL_COMPUTED,L1_FLOAT,-1.000000000,236.690521240,63.104007721,0.0,147.733261108,120.137512207,\"631T\",18,5,5,5,04,00,20,03*a038ef34\n\tsystem status\tnormal 2 27.900000 0 0\trobot status\t197.890737\t115.687001\t7.802400\t-0.859546\t-0.933418\t169.075291\t0.227000\t0.119000\n\t\n15:41:46.9\tlog_raw\tgps_raw\t#DUALANTENNAHEADINGA,USB3,0,45.5,FINESTEERING,2107,283324.900,02008000,d426,15824;SOL_COMPUTED,L1_FLOAT,-1.000000000,235.601470947,66.503868103,0.0,154.081848145,121.723312378,\"631T\",17,5,5,5,04,00,20,03*b1d66122\n\tsystem status\tnormal 2 27.900000 0 0\trobot status\t197.748728\t115.728773\t7.803100\t-0.864363\t-0.920186\t169.159833\t0.431000\t-0.191000\n\t\n15:41:47.4\tlog_raw\tgps_raw\t#DUALANTENNAHEADINGA,USB3,0,48.0,FINESTEERING,2107,283325.400,02008000,d426,15824;SOL_COMPUTED,NARROW_FLOAT,-1.000000000,247.574691772,57.258007050,0.0,263.334472656,160.580810547,\"631T\",14,8,8,7,04,00,20,23*fe321c1a\n\tsystem status\tnormal 2 27.900000 0 0\trobot status\t197.608552\t115.770934\t7.802700\t-0.846645\t-0.786369\t169.272478\t0.246000\t0.092000\n\t\n15:41:47.9\tlog_raw\tgps_raw\t#DUALANTENNAHEADINGA,USB3,0,48.0,FINESTEERING,2107,283325.900,02008000,d426,15824;SOL_COMPUTED,NARROW_FLOAT,-1.000000000,247.226425171,56.712402344,0.0,254.219528198,159.121383667,\"631T\",14,8,8,7,04,00,20,23*0ca5ab8a\n\tsystem status\tnormal 2 27.900000 0 0\trobot status\t197.468512\t115.814155\t7.802300\t-0.818285\t-0.741560\t169.351376\t0.369000\t-0.102000\n\t\n15:41:48.4\tlog_raw\tgps_raw\t\tsystem status\tnormal 2 27.900000 0 0\trobot status\t197.328854\t115.856430\t7.802000\t-0.789977\t-0.479359\t169.470018\t0.237000\t0.102000\n\t\n15:41:48.9\tlog_raw\tgps_raw\t#DUALANTENNAHEADINGA,USB3,0,49.5,FINESTEERING,2107,283326.900,02008000,d426,15824;SOL_COMPUTED,L1_FLOAT,-1.000000000,236.025100708,66.578720093,0.0,191.472290039,141.501235962,\"631T\",15,7,7,7,04,00,20,23*59a2ecb1\n\tsystem status\tnormal 2 27.900000 0 0\trobot status\t197.184762\t115.898719\t7.801800\t-0.831748\t-0.605849\t169.583780\t0.207000\t0.143000\n\t\n15:41:49.4\tlog_raw\tgps_raw\t\tsystem status\tnormal 2 27.900000 0 0\trobot status\t197.043811\t115.939828\t7.802100\t-0.874411\t-0.620436\t169.689745\t0.265000\t0.059000\n\t\n15:41:49.9\tlog_raw\tgps_raw\t#DUALANTENNAHEADINGA,USB3,0,49.5,FINESTEERING,2107,283327.900,02008000,d426,15824;SOL_COMPUTED,L1_FLOAT,-1.000000000,236.365600586,64.151107788,0.0,154.720443726,129.666244507,\"631T\",16,7,7,7,04,00,20,23*e5359168\n\tsystem status\tnormal 2 27.900000 0 0\trobot status\t196.902780\t115.981526\t7.802600\t-0.867331\t-0.776328\t169.758258\t0.275000\t0.040000\n\t\n15:41:50.4\tlog_raw\tgps_raw\t#DUALANTENNAHEADINGA,USB3,0,49.5,FINESTEERING,2107,283328.400,02000000,d426,15824;SOL_COMPUTED,L1_FLOAT,-1.000000000,233.630966187,67.887474060,0.0,142.421936035,104.273208618,\"631T\",16,7,7,7,04,00,20,23*adc689dc\n\tsystem status\tnormal 2 27.900000 0 0\trobot status\t196.761058\t116.022825\t7.801800\t-0.750648\t-1.071180\t169.858515\t0.335000\t-0.054000\n\t\n15:41:50.9\tlog_raw\tgps_raw\t\tsystem status\tnormal 2 27.900000 0 0\trobot status\t196.619455\t116.063073\t7.800700\t-0.766767\t-1.200339\t169.970662\t0.442000\t-0.208000\n\t\n15:41:51.4\tlog_raw\tgps_raw\t#INSPVAXA,USB3,0,47.5,FINESTEERING,2107,283329.450,02000000,471d,15824;INS_ALIGNMENT_COMPLETE,INS_RTKFIXED,37.37117634978,126.72305311232,7.7998,22.3000,0.0862,-0.3020,-0.0280,-0.761140788,-1.083777551,279.913760721,0.4381,0.2959,0.5691,0.1130,0.0927,0.0780,0.0968,0.1018,4.9666,0f000001,0*14477745\n\tsystem status\tnormal 2 27.900000 0 0\trobot status\t196.467447\t116.104596\t7.799800\t-0.761141\t-1.083778\t170.086239\t0.362000\t-0.099000\n\t\n15:41:51.9\tlog_raw\tgps_raw\t#DUALANTENNAHEADINGA,USB3,0,47.5,FINESTEERING,2107,283329.900,02000000,d426,15824;SOL_COMPUTED,L1_FLOAT,-1.000000000,242.466461182,68.906974792,0.0,305.866271973,174.467803955,\"631T\",16,7,7,7,04,00,20,23*70416e5a\n\tsystem status\tnormal 2 27.900000 0 0\trobot status\t196.341715\t116.139978\t7.799100\t-0.565928\t-1.102130\t170.221078\t0.416000\t-0.185000\n\t\n15:41:52.4\tlog_raw\tgps_raw\t#DUALANTENNAHEADINGA,USB3,0,45.5,FINESTEERING,2107,283330.400,02000000,d426,15824;SOL_COMPUTED,L1_FLOAT,-1.000000000,253.717498779,60.920593262,0.0,360.000000000,168.553268433,\"631T\",16,8,8,7,04,00,20,23*61124d9e\n\tsystem status\tnormal 2 27.900000 0 0\trobot status\t196.201214\t116.176846\t7.798100\t-0.490450\t-1.056663\t170.394212\t0.256000\t0.058000\n\t\n15:41:52.9\tlog_raw\tgps_raw\t\tsystem status\tnormal 2 27.900000 0 0\trobot status\t196.063617\t116.212312\t7.797500\t-0.499666\t-0.755182\t170.485971\t0.329000\t-0.041000\n\t\n15:41:53.4\tlog_raw\tgps_raw\t#DUALANTENNAHEADINGA,USB3,0,49.5,FINESTEERING,2107,283331.400,02000000,d426,15824;SOL_COMPUTED,L1_FLOAT,-1.000000000,237.639099121,66.545394897,0.0,164.585220337,123.074584961,\"631T\",15,7,7,7,04,00,20,23*2287d710\n\tsystem status\tnormal 2 27.900000 0 0\trobot status\t195.927506\t116.245468\t7.798400\t-0.593623\t-0.661216\t170.596455\t0.325000\t-0.042000\n\t\n15:41:53.9\tlog_raw\tgps_raw\t\tsystem status\tnormal 2 27.900000 0 0\trobot status\t195.790123\t116.278870\t7.800200\t-0.626746\t-0.597025\t170.660112\t0.417000\t-0.178000\n\t\n15:41:54.4\tlog_raw\tgps_raw\t#DUALANTENNAHEADINGA,USB3,0,47.5,FINESTEERING,2107,283332.400,02000000,d426,15824;SOL_COMPUTED,L1_FLOAT,-1.000000000,240.635864258,62.019580841,0.0,147.512512207,88.501113892,\"631T\",15,8,8,7,04,00,20,23*1b578ca8\n\tsystem status\tnormal 2 27.900000 0 0\trobot status\t195.687056\t116.306044\t7.801800\t-0.693124\t-0.525014\t170.661788\t0.156000\t0.006000\n\t\n15:41:54.9\tlog_raw\tgps_raw\t#DUALANTENNAHEADINGA,USB3,0,47.5,FINESTEERING,2107,283332.900,02000000,d426,15824;SOL_COMPUTED,L1_FLOAT,-1.000000000,240.870727539,61.885963440,0.0,149.317565918,88.725570679,\"631T\",15,8,8,7,04,00,20,23*f5ccc36e\n\tsystem status\tnormal 2 27.900000 0 0\trobot status\t195.536910\t116.341617\t7.803500\t-0.590606\t-0.472238\t170.823423\t0.245000\t0.069000\n\t\n15:41:55.4\tlog_raw\tgps_raw\t\tsystem status\tnormal 2 27.900000 0 0\trobot status\t195.413399\t116.372474\t7.806200\t-0.553676\t-0.333737\t170.748653\t0.336000\t-0.013000\n\t\n15:41:55.9\tlog_raw\tgps_raw\t#DUALANTENNAHEADINGA,USB3,0,47.0,FINESTEERING,2107,283333.900,02000000,d426,15824;SOL_COMPUTED,L1_FLOAT,-1.000000000,249.436477661,59.643127441,0.0,267.978637695,142.511169434,\"631T\",15,8,8,6,04,00,20,23*60a51aa1\n\tsystem status\tnormal 2 27.900000 0 0\trobot status\t195.274040\t116.405752\t7.808600\t-0.552815\t-0.398205\t170.676884\t0.284000\t-0.003000\n\t\n15:41:56.4\tlog_raw\tgps_raw\t\tsystem status\tnormal 2 27.900000 0 0\trobot status\t195.132125\t116.438540\t7.809100\t-0.730387\t-0.489733\t170.584707\t0.299000\t0.000000\n\t\n15:41:56.9\tlog_raw\tgps_raw\t\tsystem status\tnormal 2 27.900000 0 0\trobot status\t194.995838\t116.471801\t7.808500\t-0.754499\t-0.517249\t170.511574\t0.300000\t-0.003000\n\t\n15:41:57.4\tlog_raw\tgps_raw\t\tsystem status\tnormal 2 27.900000 0 0\trobot status\t194.856642\t116.507405\t7.808800\t-0.537710\t-0.683888\t170.436600\t0.302000\t-0.007000\n\t\n15:41:57.9\tlog_raw\tgps_raw\t\tsystem status\tnormal 2 27.900000 0 0\trobot status\t194.720202\t116.542041\t7.808600\t-0.456482\t-0.612371\t170.341116\t0.302000\t-0.006000\n\t\n15:41:58.4\tlog_raw\tgps_raw\t#INSPVAXA,USB3,0,48.0,FINESTEERING,2107,283336.450,02008000,471d,15824;INS_ALIGNMENT_COMPLETE,INS_RTKFIXED,37.37118062962,126.72303171077,7.8093,22.3000,0.0910,-0.2726,-0.0070,-0.431620685,-0.601507753,279.754896357,0.4400,0.2962,0.5694,0.1129,0.0927,0.0780,0.0968,0.1018,4.9757,0f000001,0*323f8ead\n\tsystem status\tnormal 2 27.900000 0 0\trobot status\t194.571733\t116.579637\t7.809300\t-0.431621\t-0.601508\t170.245104\t0.296000\t-0.009000\n\t\n15:41:58.9\t
